vi "Get Machine Name.vi"(3 "reset":bool) -> (1 "MachineName":string)   [LabVIEW 2015, in "AMC.lvlib"]
uses:
  AMC.lvlib
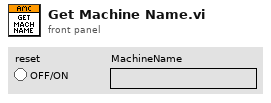
[diagram p1: front panel]
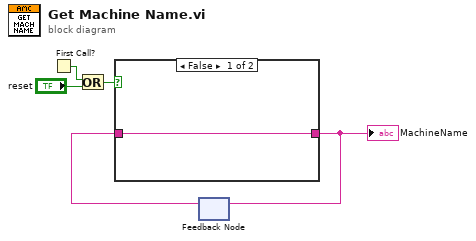
[diagram p0: block diagram]
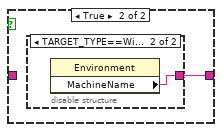
[diagram p2: hidden frame]
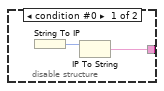
[diagram p3: hidden frame]
diagram:
  n1 = First Call?() -> (First Call?: T/F=w4:bool)
  n2 = Or(x=w4, y="reset") -> (x .or. y?=w5:bool)
  n3 = feedback #1() -> (w1:string)  [unwired: 1 in]
  n4 = case shown="False" w5 {
    tunnel: [w6 w7] -> w2
    tunnel: w1 -> [w6 _]
    frame False {
    }
    frame True {
      n5 = disable-structure shown="TARGET_TYPE==Windows" {
        disable-tunnel: [w9 w10] -> w7
        frame condition #0 {
          n6 = String To IP() -> (0:w8:u32)  [unwired: 1 out]
          n7 = IP To String(2:w8) -> (0:w9:string)  [unwired: 1 out]
        }
        frame condition #1 (active) {
          n8 = property class="Environment"() -> ("MachineName"=w10:string)  [unwired: 2 in, 2 out]
        }
      }
    }
  }
  "MachineName" <- w2
  n9 = feedback-in #1(w2) -> ()
